vi "DataTranslation_new.vi"() -> ()   [LabVIEW 2011]
doc: "This vi will take data with multiple DT boxes for an arbitrary number of channels either differentially or single ended, depending upon how you have wired the boxes up."
uses:
  Controls/DT_Cluster.ctl
  Controls/DT_Mode.ctl
  Globals/Meas_global.vi
  <userlib>/LV-Link3/PolySubVIs/DtCreateAinChan.vi
  <userlib>/LV-Link3/PolySubVIs/DtCreateCtrRateChan.vi
  <userlib>/LV-Link3/PolySubVIs/DtOLTimingSetInput.vi
  <userlib>/LV-Link3/PolySubVIs/DtOLStartNormal.vi
  <userlib>/LV-Link3/PolySubVIs/DtOLReadMultiple2D.vi
  <userlib>/LV-Link3/PolySubVIs/DtOLTriggerDigital.vi
panel:
  out "DAQ Error":errorcluster
  out "Array":T1[](array[typedef])
  out "Waveform Graph":dbl[][](graph)
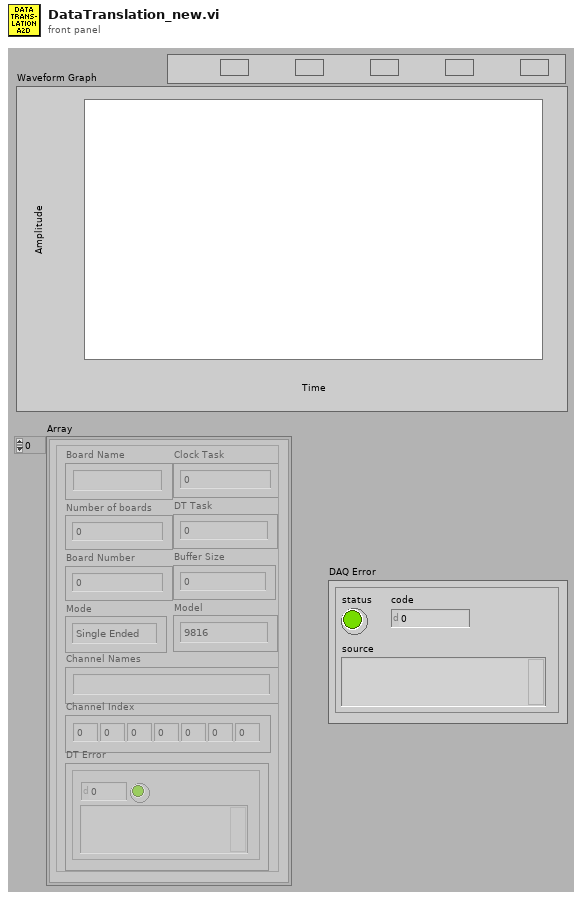
[diagram p1: front panel]
types:
  T1 = typedef "DT_Cluster.ctl" = cluster{"Board Name":string, "Number of boards":u32, "Board Number":u32, "Channel Names":string, "Channel Index":i32[], "DT Task":i32, "DT Error":errorcluster, "Mode":T2, "Buffer Size":u32, "Clock Task":i32, "Model":enum16{"9816", "9836", "9853"}}
  T2 = typedef "DT_Mode.ctl" = enum16{"Single Ended", "Differential"}
  T3 = typedef "Trigger_Mode.ctl" = enum16{"Free Running", "Start on Trigger", "Trigger Every Block", "Trigger Every Sample"}
  T4 = enum32{"Internal Clock", "External Clock", "No Timing"}
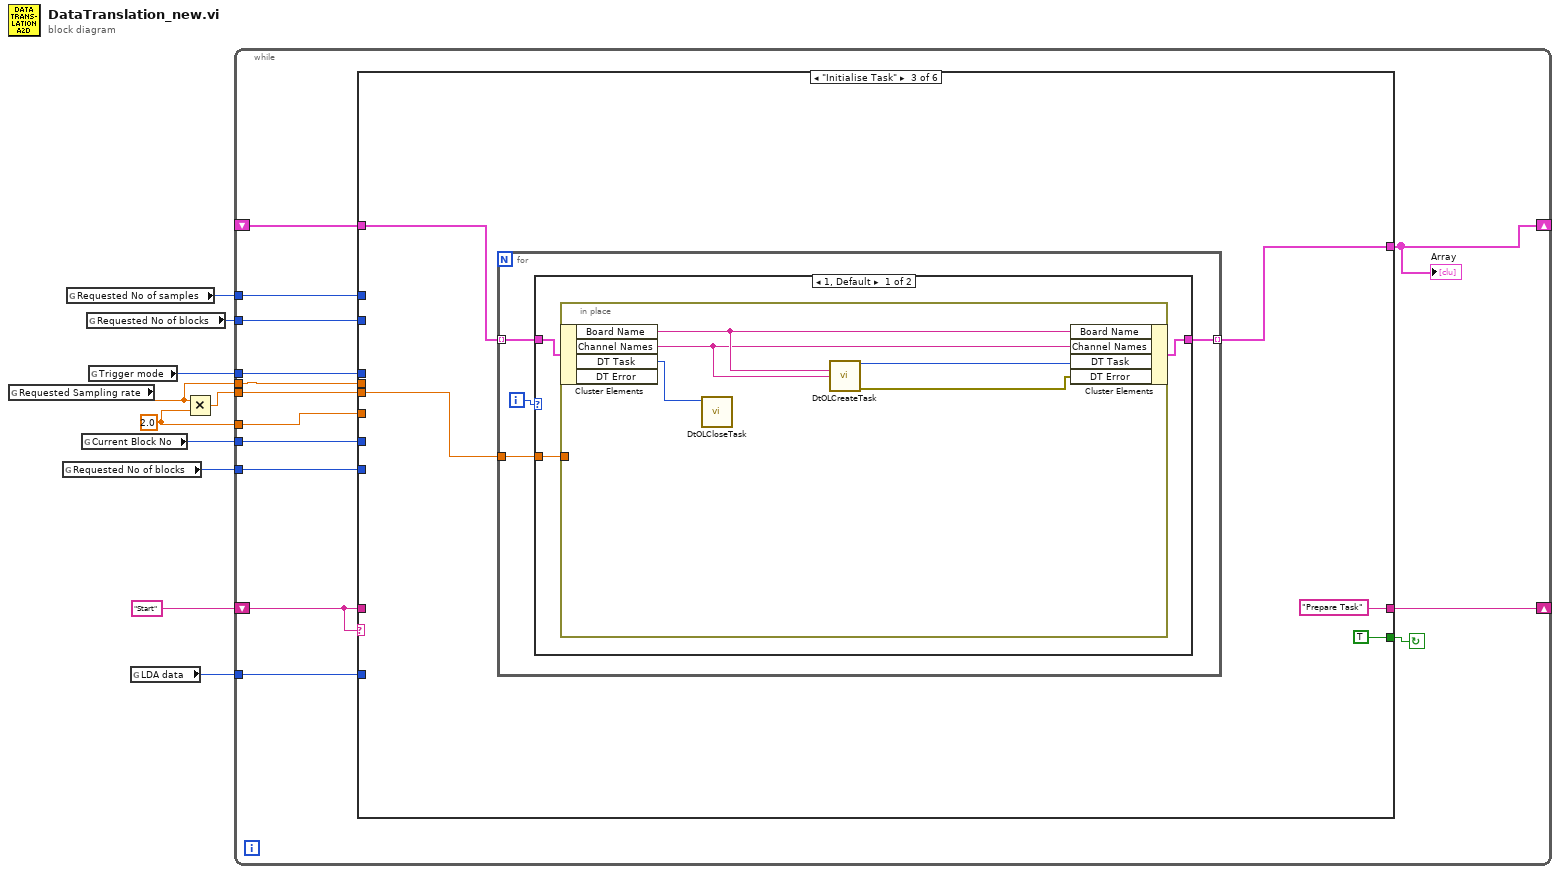
[diagram p0: block diagram]
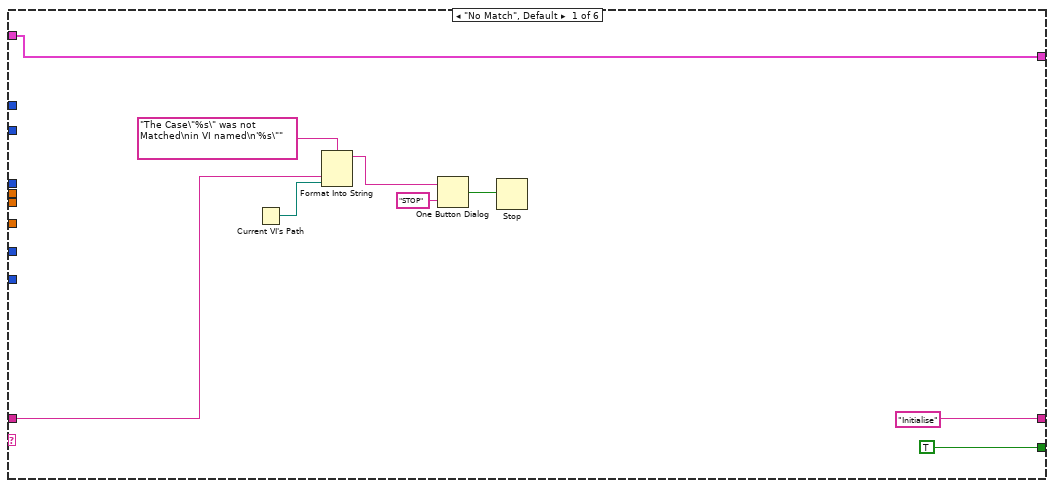
[diagram p2: hidden frame]
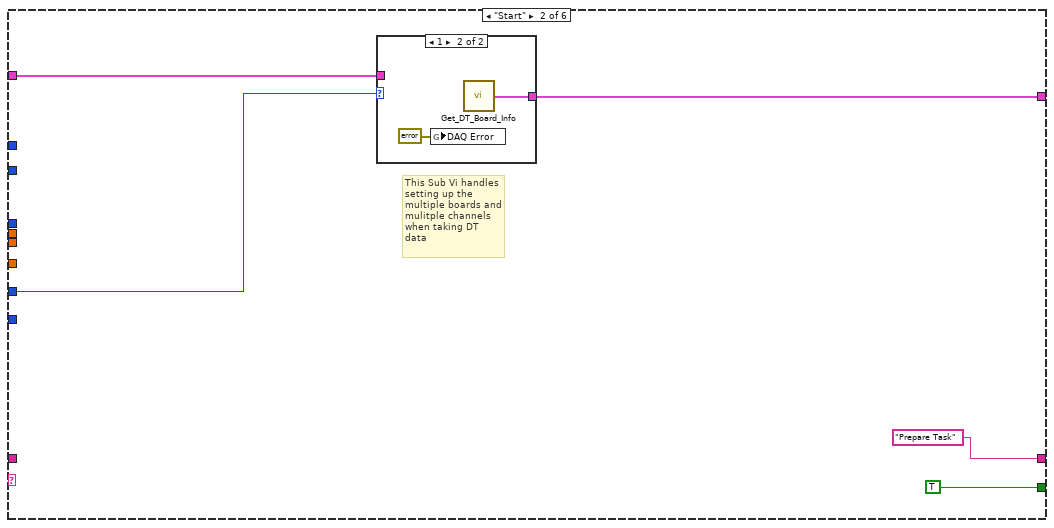
[diagram p3: hidden frame]
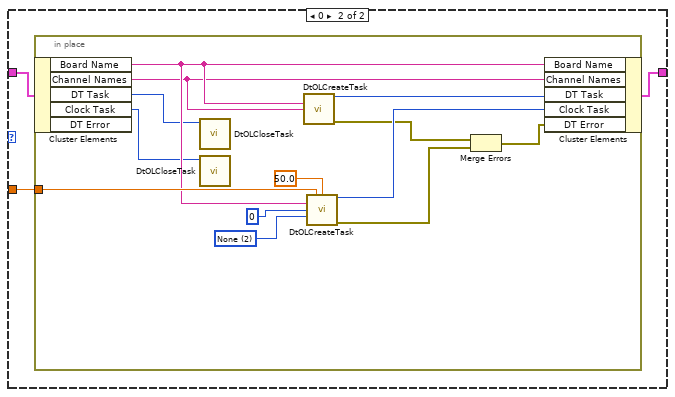
[diagram p5: hidden frame]
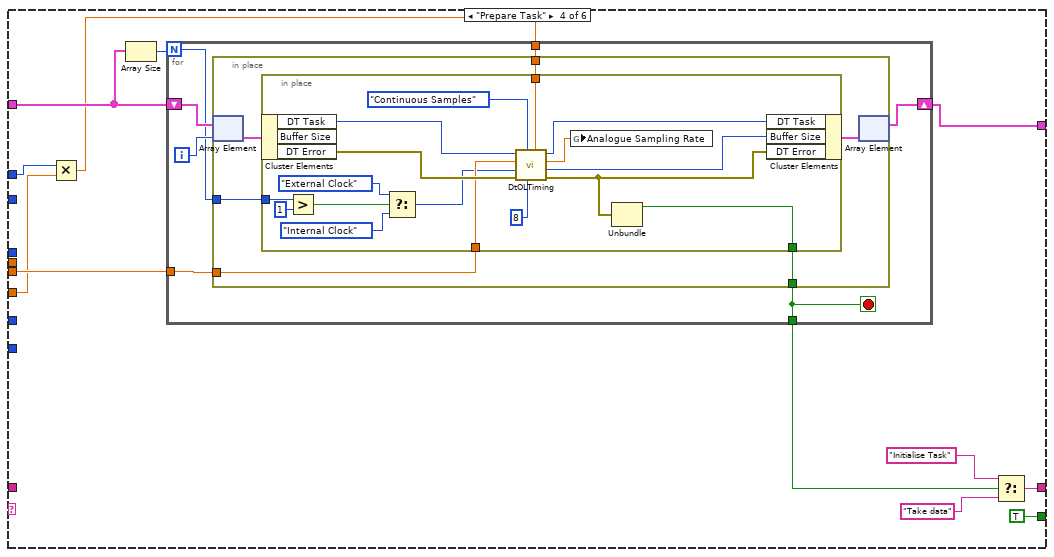
[diagram p6: hidden frame]
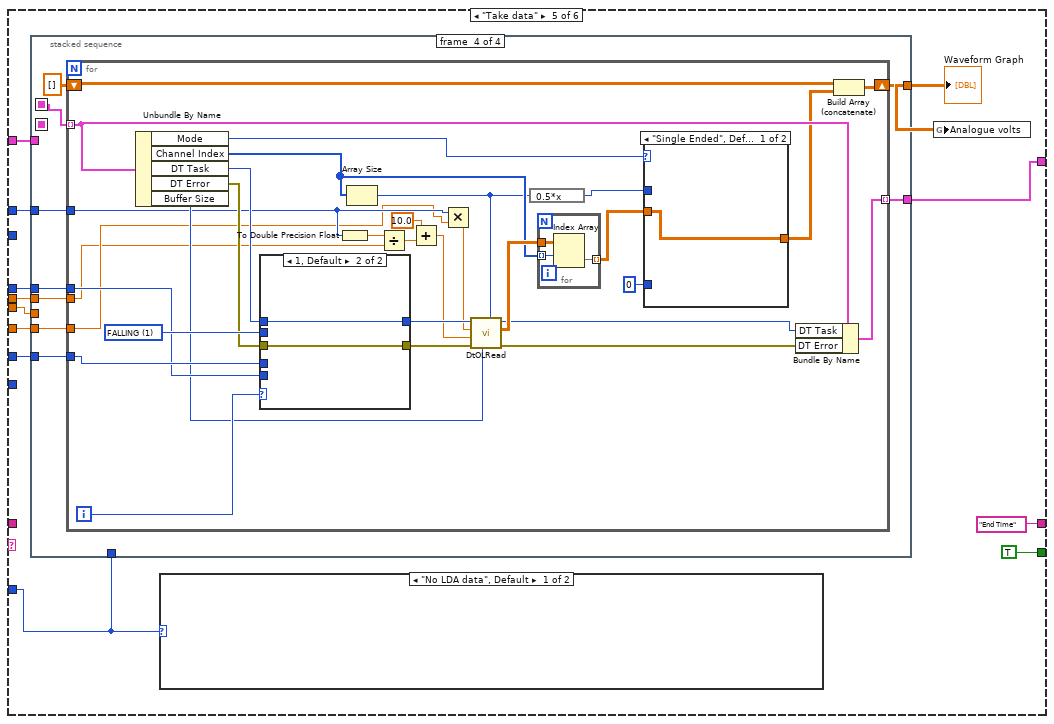
[diagram p7: hidden frame]
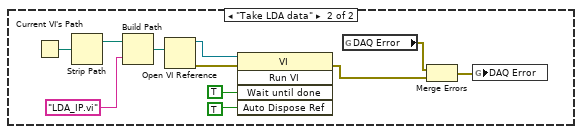
[diagram p8: hidden frame]
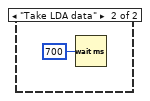
[diagram p10: hidden frame]
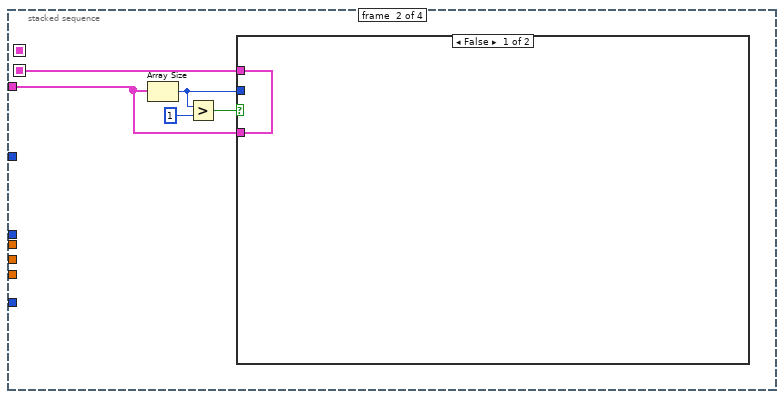
[diagram p11: hidden frame]
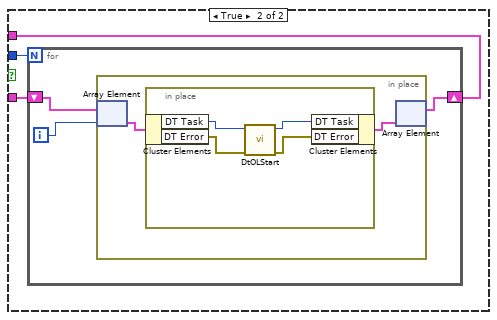
[diagram p12: hidden frame]
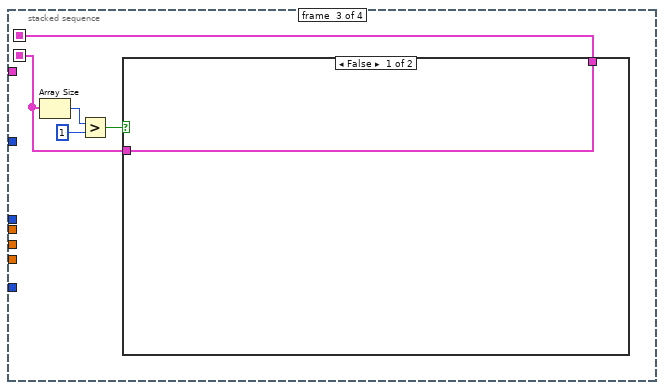
[diagram p13: hidden frame]
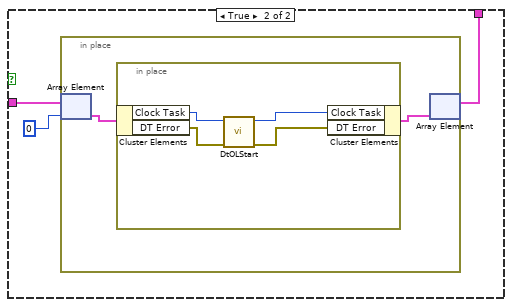
[diagram p14: hidden frame]
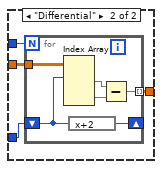
[diagram p15: hidden frame]
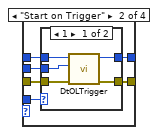
[diagram p18: hidden frame]
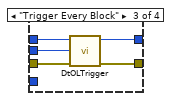
[diagram p20: hidden frame]
diagram:
  w3 = 2.0 ("y")
  n1 = global read "Meas_global.vi" "Requested Sampling rate"() -> (w2:dbl)
  n2 = global read "Meas_global.vi" "Requested No of blocks"() -> (w1:i32)
  n3 = global read "Meas_global.vi" "Requested No of samples"() -> (w9:i32)
  n4 = global read "Meas_global.vi" "Current Block No"() -> (w7:i32)
  n5 = global read "Meas_global.vi" "Requested No of blocks"() -> (w6:i32)
  n6 = global read "Meas_global.vi" "Trigger mode"() -> (w8:T3)
  n7 = global read "Meas_global.vi" "LDA data"() -> (w5:enum16{"No LDA data", "Take LDA data"})
  n8 = Multiply(x=w2, y=w3) -> (x*y=w4:dbl)
  n9 = while {
    shift-left: "Start" -> [w23]
    shift-right: [w24] -> _
    tunnel: w4 -> [w22]
    tunnel: w9 -> [w21]
    tunnel: w7 -> [w20]
    tunnel: w8 -> [w18]
    tunnel: w6 -> [w17]
    shift-right: [w16] -> _
    shift-left: _ -> [w15]
    tunnel: w5 -> [w14]
    tunnel: w3 -> [w13]
    tunnel: w2 -> [w12]
    tunnel: w1 -> [w11]
    stop <- w19 continue-if-true
    n10 = case shown="\"Initialise Task\"" w23 {
      tunnel: ["Initialise" "Prepare Task" "Prepare Task" w83 "End Time" "" ("f")] -> w24
      tunnel: w23 -> [w29 _ _ _ _ _]
      tunnel: w22 -> [_ _ w44 w79 w117 _]
      tunnel: w21 -> [_ _ _ w77 w127 _]
      tunnel: w20 -> [_ w34 _ _ w125 w262]
      tunnel: [TRUE TRUE TRUE TRUE TRUE FALSE] -> w19
      tunnel: w18 -> [_ _ _ _ w124 _]
      tunnel: w17 -> [_ _ _ _ _ _]
      tunnel: w15 -> [w25 w36 w42 w78 w123 w266]
      tunnel: [w25 w37 w43 w80 w122 w265] -> w16
      tunnel: w14 -> [_ _ _ _ w118 _]
      tunnel: w13 -> [_ _ _ w76 w120 _]
      tunnel: w12 -> [_ _ _ _ w119 _]
      tunnel: w11 -> [_ _ _ _ _ w263]
      frame "No Match", Default {
        n11 = Current VI's Path() -> (path=w28:path)
        n12 = Format Into String(format string="The Case\"%s\" was not Matched\nin VI named\n'%s\"" ("Format String"), w29, w28) -> (resulting string=w32:string)  [unwired: 2 in, 1 out]
        n13 = One Button Dialog(message=w32, button name ("OK")="STOP") -> (true=w30:bool)
        n14 = Stop(stop? (T)=w30) -> ()
      }
      frame "Start" {
        # "This Sub Vi handles setting up the multiple boards and mulitple channels when taking DT data"
        n15 = case shown="1" w34 {
          tunnel: [w39 w41] -> w37
          tunnel: w36 -> [w39 _]
          frame 2, Default {
          }
          frame 1 {
            n16 = global write "Meas_global.vi" "DAQ Error"(errorcluster {"status"=FALSE, "code"=0, "source"=""} ("DAQ Error")) -> ()
            n17 = call "Get_DT_Board_Info.vi"() -> ("DT Cluster Array"=w41:T1[])  [unwired: 5 in]
          }
        }
      }
      frame "Initialise Task" {
        n18 = for {
          tunnel: w42 -> [w50] mode=indexing
          tunnel: w44 -> [w49]
          tunnel: [w48] -> w43 mode=indexing
          i -> [w47]
          n19 = case shown="1, Default" w47 {
            tunnel: w50 -> [w53 w61]
            tunnel: w49 -> [w52 w60]
            tunnel: [w51 w59] -> w48
            frame 1, Default {
              n20 = in-place {
                in-place-border: w52 -> [_]
                n21 = in-place-cluster #1(w53) -> ("Board Name"=w58:string, "Channel Names"=w55:string, "DT Task"=w54:i32)  [unwired: 1 out]
                n22 = call <userlib>:"DtOLCloseTask.vi"("Task in"=w54) -> ()  [unwired: 10 in, 1 out]
                n23 = call-poly <userlib>:"DtOLCreateTask.vi"("Board Name"=w58, "Channel"=w55) -> ("Task out"=w57:i32, "error out"=w56:errorcluster)  [unwired: 11 in, 1 out]
                n24 = in-place-cluster #1("Board Name"=w58, "Channel Names"=w55, "DT Task"=w57, "DT Error"=w56) -> (w51:T1)
              }
            }
            frame 0 {
              n25 = in-place {
                in-place-border: w60 -> [w71]
                w74 = 2 items=["LowLevel", "HighLevel", "None"] ("Gate Type")
                n26 = in-place-cluster #2(w61) -> ("Board Name"=w69:string, "Channel Names"=w64:string, "DT Task"=w63:i32, "Clock Task"=w62:i32)  [unwired: 1 out]
                n27 = call <userlib>:"DtOLCloseTask.vi"("Task in"=w63) -> ()  [unwired: 10 in, 1 out]
                n28 = call <userlib>:"DtOLCloseTask.vi"("Task in"=w62) -> ()  [unwired: 10 in, 1 out]
                n29 = call-poly <userlib>:"DtOLCreateTask.vi"("Board Name"=w69, "Channel"=w64) -> ("Task out"=w68:i32, "error out"=w66:errorcluster)  [unwired: 11 in, 1 out]
                n30 = call-poly <userlib>:"DtOLCreateTask.vi"("Requested\nFrequency (Hz)"=w71, "Duty Cycle"=50.0, "Board Name"=w69, "Counter Num"=u32 0, "Gate Type"=w74) -> ("Task out"=w67:i32, "error out"=w70:errorcluster)  [unwired: 8 in, 1 out]
                n31 = Merge Errors(w66, w70) -> (w65:errorcluster)
                n32 = in-place-cluster #2("Board Name"=w69, "Channel Names"=w64, "DT Task"=w68, "Clock Task"=w67, "DT Error"=w65) -> (w59:T1)
              }
            }
          }
        }
      }
      frame "Prepare Task" {
        n33 = Multiply(x=w77, y=w76) -> (x*y=w75:dbl)
        n34 = Array Size(array=w78) -> (size(s)=w82:i32)
        n35 = for {
          N: w82 -> [w87]
          shift-right: [w90] -> w80
          shift-left: w78 -> [w92]
          tunnel: [w93] -> w81
          tunnel: w79 -> [w89]
          tunnel: w75 -> [w88]
          i -> [w91]
          stop <- w93 stop-if-true
          n36 = in-place {
            in-place-border: [w99] -> w93
            in-place-border: w89 -> [w96]
            in-place-border: w88 -> [w95]
            in-place-border: w87 -> [w94]
            n37 = in-place-array #3(w92, w91) -> (w98:T1)
            n38 = in-place {
              in-place-border: [w108] -> w99
              in-place-border: w96 -> [w107]
              in-place-border: w95 -> [w106]
              in-place-border: w94 -> [w105]
              n39 = in-place-cluster #4(w98) -> ("DT Task"=w114:i32, "DT Error"=w113:errorcluster)  [unwired: 1 out]
              n40 = Greater?(x=w105, y=1) -> (0:w103:bool)
              n41 = Select(t=T4."External Clock" ("Timing"), s=w103, f=T4."Internal Clock" ("Timing")) -> (s? t:f=w100:T4)
              n42 = call-poly <userlib>:"DtOLTiming.vi"("Samples Per Channel"=w106, "Num Buffers"=u32 8, "Sample Mode"=enum16{"Finite Samples", "Continuous Samples"}."Continuous Samples", "error in (no error)"=w113, "Timing"=w100, "Sample Freq (Hz)"=w107, "Task in"=w114) -> ("error out"=w109:errorcluster, "Buffer Size"=w112:u32, "Actual Sample Freq"=w115:dbl, "Task out"=w111:i32)  [unwired: 1 in]
              n43 = global write "Meas_global.vi" "Analogue Sampling Rate"(w115) -> ()
              n44 = Unbundle(w109) -> ("status"=w108:bool)  [unwired: 2 out]
              n45 = in-place-cluster #4("DT Task"=w111, "Buffer Size"=w112, "DT Error"=w109) -> (w97:T1)
            }
            n46 = in-place-array #3(w97) -> (w90:T1[])  [unwired: 1 out]
          }
        }
        n47 = Select(t="Initialise Task", s=w81, f="Take data") -> (s? t:f=w83:string)
      }
      frame "Take data" {
        n48 = stacked-sequence {
          seq-local: [_ w146 _ _] -> [_ _ w161 _]
          seq-local: [_ _ w164 _] -> [_ _ _ w175]
          tunnel: w127 -> [_ _ _ w183]
          tunnel: w125 -> [_ _ _ w182]
          tunnel: w124 -> [_ _ _ w181]
          tunnel: w123 -> [_ w145 _ _]
          tunnel: [_ _ _ w180] -> w122
          tunnel: [_ _ _ w178] -> w121
          tunnel: w120 -> [_ _ _ w177]
          tunnel: w119 -> [_ _ _ w176]
          tunnel: w118 -> [w140 _ _ _]
          tunnel: w117 -> [_ _ _ _]
          frame #0 {
            n49 = case shown="\"No LDA data\", Default" w140 {
              frame "No LDA data", Default {
              }
              frame "Take LDA data" {
                n50 = Wait (ms)(milliseconds to wait=u32 700) -> ()  [unwired: 1 out]
              }
            }
          }
          frame #1 {
            n51 = Array Size(array=w145) -> (size(s)=w144:i32)
            n52 = Greater?(x=w144, y=1) -> (0:w142:bool)
            n53 = case shown="False" w142 {
              tunnel: [w147 w150] -> w146
              tunnel: w145 -> [w147 w149]
              tunnel: w144 -> [_ w148]
              frame False {
              }
              frame True {
                n54 = for {
                  N: w148 -> [_]
                  shift-right: [w151] -> w150
                  shift-left: w149 -> [w152]
                  i -> [w153]
                  n55 = in-place {
                    n56 = in-place-array #5(w152, w153) -> (w155:T1)
                    n57 = in-place {
                      n58 = in-place-cluster #6(w155) -> ("DT Task"=w159:i32, "DT Error"=w158:errorcluster)
                      n59 = call-poly <userlib>:"DtOLStart.vi"("error in (no error)"=w158, "Task in"=w159) -> ("error out"=w157:errorcluster, "Task out"=w156:i32)  [unwired: 8 in]
                      n60 = in-place-cluster #6("DT Task"=w156, "DT Error"=w157) -> (w154:T1)
                    }
                    n61 = in-place-array #5(w154) -> (w151:T1[])  [unwired: 1 out]
                  }
                }
              }
            }
          }
          frame #2 {
            n62 = Array Size(array=w161) -> (size(s)=w163:i32)
            n63 = Greater?(x=w163, y=1) -> (0:w160:bool)
            n64 = case shown="False" w160 {
              tunnel: [w165 w167] -> w164
              tunnel: w161 -> [w165 w166]
              frame False {
              }
              frame True {
                n65 = in-place {
                  n66 = in-place-array #7(w166, 0) -> (w170:T1)
                  n67 = in-place {
                    n68 = in-place-cluster #8(w170) -> ("Clock Task"=w173:i32, "DT Error"=w174:errorcluster)
                    n69 = call-poly <userlib>:"DtOLStart.vi"("error in (no error)"=w174, "Task in"=w173) -> ("error out"=w171:errorcluster, "Task out"=w172:i32)  [unwired: 8 in]
                    n70 = in-place-cluster #8("Clock Task"=w172, "DT Error"=w171) -> (w169:T1)
                  }
                  n71 = in-place-array #7(w169) -> (w167:T1[])  [unwired: 1 out]
                }
              }
            }
          }
          frame #3 {
            n72 = for {
              tunnel: w183 -> [w188]
              tunnel: w182 -> [w212]
              tunnel: w181 -> [w211]
              tunnel: w175 -> [w207] mode=indexing
              tunnel: [w206] -> w180 mode=indexing
              shift-right: [w203] -> w178
              shift-left: dbl[][] [] -> [w202]
              tunnel: w177 -> [w187]
              tunnel: w176 -> [w185]
              i -> [w197]
              w213 = 1 items=["RISING", "FALLING"] ("External Trigger Polarity")
              n73 = Unbundle By Name(w207) -> ("Mode"=w194:T2, "Channel Index"=w204:i32[], "DT Task"=w210:i32, "DT Error"=w209:errorcluster, "Buffer Size"=w190:u32)
              n74 = case shown="1, Default" w197 {
                tunnel: [w232 w256] -> w214
                tunnel: w213 -> [w231 _]
                tunnel: w212 -> [w230 _]
                tunnel: w211 -> [w229 _]
                tunnel: w210 -> [w228 w256]
                tunnel: w209 -> [w227 w255]
                tunnel: [w226 w255] -> w208
                frame 0 {
                  n75 = case shown="\"Trigger Every Sample\"" w229 {
                    tunnel: [w234 w238 w250 w254] -> w232
                    tunnel: w228 -> [w234 w239 w252 w254]
                    tunnel: w230 -> [_ w240 _ _]
                    tunnel: w231 -> [_ w237 w251 _]
                    tunnel: w227 -> [w233 w236 w249 w253]
                    tunnel: [w233 w235 w248 w253] -> w226
                    frame "Free Running" {
                    }
                    frame "Start on Trigger" {
                      n76 = case shown="1" w240 {
                        tunnel: w239 -> [w245 w247]
                        tunnel: w236 -> [w244 w246]
                        tunnel: [w242 w247] -> w238
                        tunnel: [w243 w246] -> w235
                        tunnel: w237 -> [w241 _]
                        frame 1 {
                          n77 = call-poly <userlib>:"DtOLTrigger.vi"("error in (no error)"=w244, "External Trigger Polarity"=w241, "Task in"=w245) -> ("error out"=w243:errorcluster, "Task out"=w242:i32)  [unwired: 7 in]
                        }
                        frame 2, Default {
                        }
                      }
                    }
                    frame "Trigger Every Block" {
                      n78 = call-poly <userlib>:"DtOLTrigger.vi"("error in (no error)"=w249, "External Trigger Polarity"=w251, "Task in"=w252) -> ("error out"=w248:errorcluster, "Task out"=w250:i32)  [unwired: 7 in]
                    }
                    frame "Trigger Every Sample" {
                    }
                  }
                }
                frame 1, Default {
                }
              }
              n79 = To Double Precision Float(number=w188) -> (double precision float=w201:dbl)
              n80 = Array Size(array=w204) -> (size(s)=w192:i32)
              n81 = Divide(x=w201, y=w185) -> (x/y=w200:dbl)
              n82 = Add(x=10.0, y=w200) -> (x+y=w198:dbl)
              n83 = Multiply(x=w188, y=w187) -> (x*y=w186:dbl)
              n84 = call-poly <userlib>:"DtOLRead.vi"("Number Chan to Read"=w192, "Buffer size"=w190, "error in (no error)"=w208, "Timeout"=w198, "Samples Per Channel"=w186, "Task in"=w214) -> ("error out"=w189:errorcluster, "2D Data out"=w205:dbl[][], "Task out"=w196:i32)  [unwired: 1 in, 2 out]
              n85 = expression code="0.5*x"(w192) -> (w191:i32)
              n86 = for {
                tunnel: w204 -> [w259] mode=indexing
                tunnel: w205 -> [w258]
                tunnel: [w257] -> w184 mode=indexing
                n87 = Index Array(array=w258, index (row)=w259) -> (element=w257:dbl[])  [unwired: 1 in]
              }
              n88 = case shown="\"Single Ended\", Default" w194 {
                tunnel: w184 -> [w215 w219]
                tunnel: [w215 w218] -> w195
                tunnel: 0 ("size(s)") -> [_ w217]
                tunnel: w191 -> [_ w216]
                frame "Single Ended", Default {
                }
                frame "Differential" {
                  n89 = for {
                    N: w216 -> [_]
                    tunnel: w219 -> [w225]
                    shift-right: [w224] -> _
                    shift-left: w217 -> [w223]
                    tunnel: [w221] -> w218 mode=indexing
                    n90 = Index Array(array=w225, index (row) #1=w223) -> (element #1=w220:dbl[], element #2=w222:dbl[])  [unwired: 3 in]
                    n91 = expression code="x+2"(w223) -> (w224:i32)
                    n92 = Subtract(x=w220, y=w222) -> (x-y=w221:dbl[])
                  }
                }
              }
              n93 = Bundle By Name(cluster=w207, "DT Task"=w196, "DT Error"=w189) -> (w206:T1)
              n94 = Build Array (concatenate)(w202, w195) -> (w203:dbl[][])
            }
          }
        }
        "Waveform Graph" <- w121
        n95 = case shown="\"No LDA data\", Default" w118 {
          frame "No LDA data", Default {
          }
          frame "Take LDA data" {
            n96 = Current VI's Path() -> (path=w133:path)
            n97 = Strip Path(path=w133) -> (stripped path=w129:path)  [unwired: 1 out]
            n98 = Build Path(base path=w129, name or relative path="LDA_IP.vi") -> (appended path=w134:path)
            n99 = Open VI Reference(vi path=w134) -> (vi reference=w137:refnum<vi>, error out=w138:errorcluster)  [unwired: 5 in]
            n100 = invoke class="VI" method="Run VI"(reference=w137, error in=w138, "Wait until done"=TRUE ("Wait Until Done"), "Auto Dispose Ref"=TRUE ("Wait until done")) -> (error out=w131:errorcluster)  [unwired: 1 in, 4 out]
            n101 = global read "Meas_global.vi" "DAQ Error"() -> (w132:errorcluster)
            n102 = Merge Errors(w132, w131) -> (w130:errorcluster)
            n103 = global write "Meas_global.vi" "DAQ Error"(w130) -> ()
          }
        }
        n104 = global write "Meas_global.vi" "Analogue volts"(w121) -> ()
      }
      frame "End Time" {
        n105 = Equal?(x=w262, y=w263) -> (x = y?=w260:bool)
        n106 = case shown="False" w260 {
          tunnel: w266 -> [w269 w271]
          tunnel: [w269 w270] -> w265
          frame False {
          }
          frame True {
            n107 = for {
              tunnel: w271 -> [w274] mode=indexing
              tunnel: [w273] -> w270 mode=indexing
              i -> [w272]
              n108 = case shown="1, Default" w272 {
                tunnel: w274 -> [w276 w282]
                tunnel: [w275 w281] -> w273
                frame 1, Default {
                  n109 = in-place {
                    n110 = in-place-cluster #9(w276) -> ("DT Task"=w280:i32, "DT Error"=w279:errorcluster)
                    n111 = call <userlib>:"DtOLCloseTask.vi"("Error in"=w279, "Task in"=w280) -> ("Error Out"=w278:errorcluster)  [unwired: 9 in]
                    n112 = in-place-cluster #9("DT Task"=0, "DT Error"=w278) -> (w275:T1)
                  }
                }
                frame 0 {
                  n113 = in-place {
                    n114 = in-place-cluster #10(w282) -> ("DT Task"=w288:i32, "DT Error"=w287:errorcluster, "Clock Task"=w285:i32)
                    n115 = call <userlib>:"DtOLCloseTask.vi"("Task in"=w285) -> ("Error Out"=w290:errorcluster)  [unwired: 10 in]
                    n116 = call <userlib>:"DtOLCloseTask.vi"("Error in"=w287, "Task in"=w288) -> ("Error Out"=w286:errorcluster)  [unwired: 9 in]
                    n117 = Merge Errors(w286, w290) -> (w289:errorcluster)
                    n118 = in-place-cluster #10("DT Task"=0, "DT Error"=w289, "Clock Task"=0) -> (w281:T1)
                  }
                }
              }
            }
          }
        }
        n119 = global read "Meas_global.vi" "DAQ Error"() -> (w261:errorcluster)
        n120 = for {
          tunnel: w265 -> [w294] mode=indexing
          shift-right: [w291] -> w264
          shift-left: w261 -> [w292]
          n121 = Unbundle By Name(w294) -> ("DT Error"=w293:errorcluster)
          n122 = Merge Errors(w292, w293) -> (w291:errorcluster)
        }
        "DAQ Error" <- w264
        n123 = global write "Meas_global.vi" "DAQ Error"(w264) -> ()
      }
    }
    "Array" <- w16
  }
